vi "ApplyScatterVector.vi"(10 "Scatter Coordinates (Spherical)":cluster{"R":dbl, "Theta":dbl, "Phi":dbl}={"R"=nan, "Theta"=nan, "Phi"=nan}, 11 "Old Velocity Vector (X,Y,Z)":cluster{"X":dbl, "Y":dbl, "Z":dbl}) -> (3 "New Velocity Vector (X,Y,Z)":cluster{"X":dbl, "Y":dbl, "Z":dbl})   [LabVIEW 2019]
uses:
  <vilib>/Analysis/NI_AALPro.lvlib
panel:
  out "Oy":cluster{"X":dbl, "Y":dbl, "Z":dbl}
  out "Oz":cluster{"X":dbl, "Y":dbl, "Z":dbl}
  out "Ox":cluster{"X":dbl, "Y":dbl, "Z":dbl}={"X"=nan, "Y"=nan, "Z"=nan}
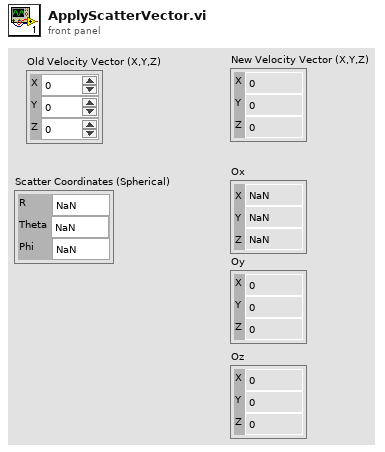
[diagram p1: front panel]
types:
  T1 = cluster{"Cross Product[0]":dbl, "Cross Product[1]":dbl, "Cross Product[2]":dbl}
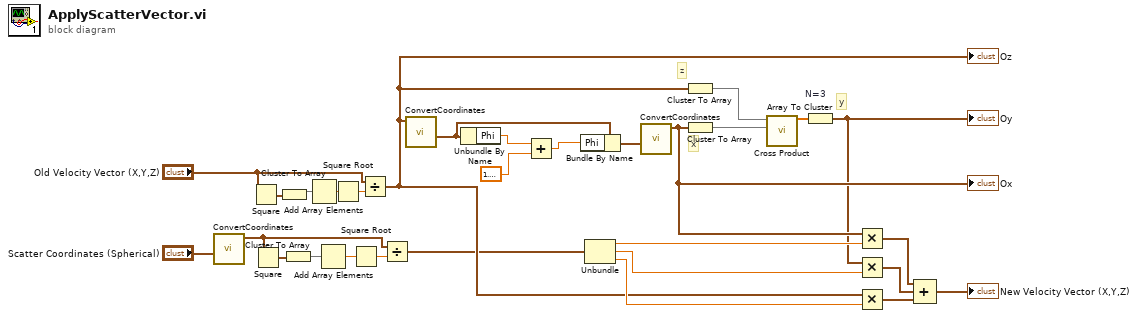
[diagram p0: block diagram]
diagram:
  # "y"
  # "z"
  # "x"
  n1 = call "ConvertCoordinates.vi"("Spherical Coordinates In"="Scatter Coordinates (Spherical)") -> ("XYZ Coordinates Out"=w5:cluster{"X":dbl, "Y":dbl, "Z":dbl})  [unwired: 7 in, 3 out]
  n2 = Square(x="Old Velocity Vector (X,Y,Z)") -> (x^2=w13:cluster{"X":dbl, "Y":dbl, "Z":dbl})
  n3 = Square(x=w5) -> (x^2=w6:cluster{"X":dbl, "Y":dbl, "Z":dbl})
  n4 = Cluster To Array(cluster=w13) -> (array=w12:dbl[])
  n5 = Cluster To Array(cluster=w6) -> (array=w7:dbl[])
  n6 = Add Array Elements(numeric array=w12) -> (sum=w11:dbl)
  n7 = Add Array Elements(numeric array=w7) -> (sum=w8:dbl)
  n8 = Square Root(x=w11) -> (sqrt(x)=w3:dbl)
  n9 = Square Root(x=w8) -> (sqrt(x)=w2:dbl)
  n10 = Divide(x="Old Velocity Vector (X,Y,Z)", y=w3) -> (x/y=w9:cluster{"X":dbl, "Y":dbl, "Z":dbl})
  "Oz" <- w9
  n11 = Divide(x=w5, y=w2) -> (x/y=w4:cluster{"X":dbl, "Y":dbl, "Z":dbl})
  n12 = call "ConvertCoordinates.vi"("XYZ Coordinates In"=w9) -> ("Spherical Coordinates Out"=w28:cluster{"R":dbl, "Theta":dbl, "Phi":dbl})  [unwired: 7 in, 3 out]
  n13 = Unbundle By Name(w28) -> ("Phi"=w30:dbl)
  n14 = Add(x=w30, y=1.5707963267948966) -> (x+y=w27:dbl)
  n15 = Bundle By Name(cluster=w28, "Phi"=w27) -> (w26:cluster{"R":dbl, "Theta":dbl, "Phi":dbl})
  n16 = Unbundle(w4) -> ("X"=w22:dbl, "Y"=w19:dbl, "Z"=w20:dbl)
  n17 = call "ConvertCoordinates.vi"("Spherical Coordinates In"=w26) -> ("XYZ Coordinates Out"=w21:cluster{"X":dbl, "Y":dbl, "Z":dbl})  [unwired: 7 in, 3 out]
  "Ox" <- w21
  n18 = Cluster To Array(cluster=w9) -> (array=w24:dbl[])
  n19 = Cluster To Array(cluster=w21) -> (array=w25:dbl[])
  n20 = call <vilib>:"Cross Product.vi"("B Vector"=w25, "A Vector"=w24) -> ("Cross Product"=w23:dbl[])  [unwired: 8 in, 1 out]
  n21 = Array To Cluster "N=3"(array=w23) -> (cluster=w18:T1)
  "Oy" <- w18
  n22 = Multiply(x=w21, y=w22) -> (x*y=w15:cluster{"X":dbl, "Y":dbl, "Z":dbl})
  n23 = Multiply(x=w18, y=w19) -> (x*y=w16:T1)
  n24 = Multiply(x=w9, y=w20) -> (x*y=w17:cluster{"X":dbl, "Y":dbl, "Z":dbl})
  n25 = Compound Arithmetic op=ADD(w15, w16, w17) -> (→"New Velocity Vector (X,Y,Z)":cluster{dbl, dbl, dbl})
